vi "EX2.vi"() -> ()   [LabVIEW 2018]
panel:
  out "LED":bool
  in  "SWITCH":bool
  out "date string":string
  out "time string":string
  # "EX2 - TP0"
  # "Mekni Marwen 2ème Année Génie Electrique"
  # "Led control with a switch"
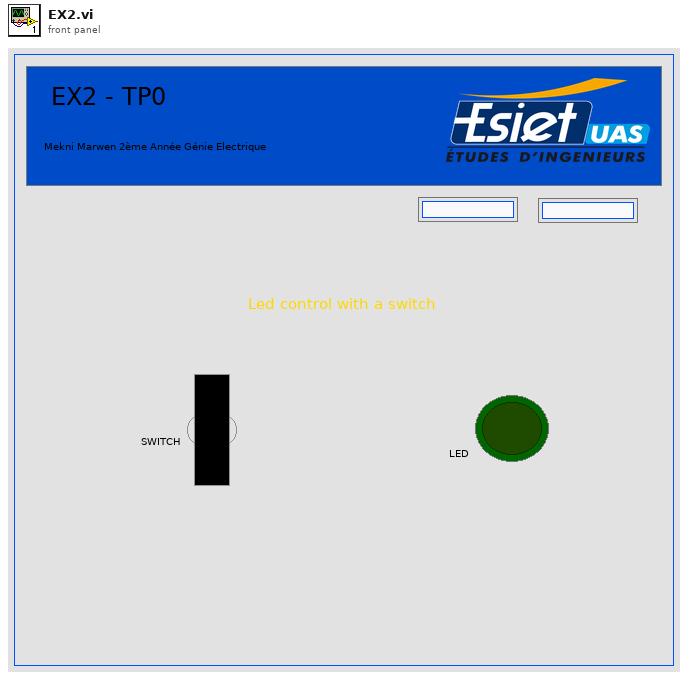
[diagram p1: front panel]
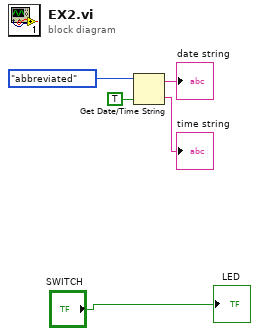
[diagram p0: block diagram]
diagram:
  n1 = Get Date/Time String(date format (0)=enum16{"short", "long", "abbreviated"}."abbreviated", want seconds? (F)=TRUE) -> (date string=→"date string":string, time string=→"time string":string)  [unwired: 1 in]
  "LED" <- "SWITCH"
